vi "Multi-channel FFT(lvgpu).vi"() -> ()   [LabVIEW 2020]
doc: "Computes the 1D FFT of multiple signals simultaneously using a GPU device."
uses:
  subVIs/Channel Data Type.ctl
  <vilib>/addons/lvgpu/lvcufft/CUFFT Type (cufftType).ctl
  <vilib>/addons/lvgpu/lvcufft/Create 1D FFT Plan.vi
  <vilib>/addons/lvgpu/lvcuda/CUDA CSG Device Ptr/Download 2D Data.vi
  <vilib>/addons/lvgpu/lvcufft/Complex FFT (CSG).vi
  <vilib>/addons/lvgpu/lvcuda/CUDA CSG Device Ptr/Upload 2D Data.vi
  <vilib>/addons/lvgpu/lvcufft.lvlib
  <vilib>/addons/lvgpu/lvcuda.lvlib
  subVIs/Multi-channel FFT.lvlib
  <vilib>/ptbypt/NI_PtbyPt.lvlib
  <vilib>/addons/lvgpu/lvcuda/CUDA CSG Device Ptr/CUDA CSG Device Ptr.lvclass
panel:
  in  "Execution Info":T1(tab)
  out "Current Channel":sgl[](graph)
  out "Current Spectrum":sgl[][](graph)
  out "Error Status":errorcluster
  out "CUDA Version":string
  out "CUDA Display Driver Version":string
  out "GPU Device Name":string
  in  "Channel Data":T2 items=["Pulsing Sine Wave", "Fixed Sine Wave", "Drifting Sine Wave"]
  out "GPU Exec Time":dbl format="%#_2p"
  in  "Device ID":i32 min=0 max=0
  out "Intensity Graph (dB)":sgl[][](graph)
  in  "stop":bool
  in  "Samples / channel":i32=1024
  in  "Number of channels":i32=1024
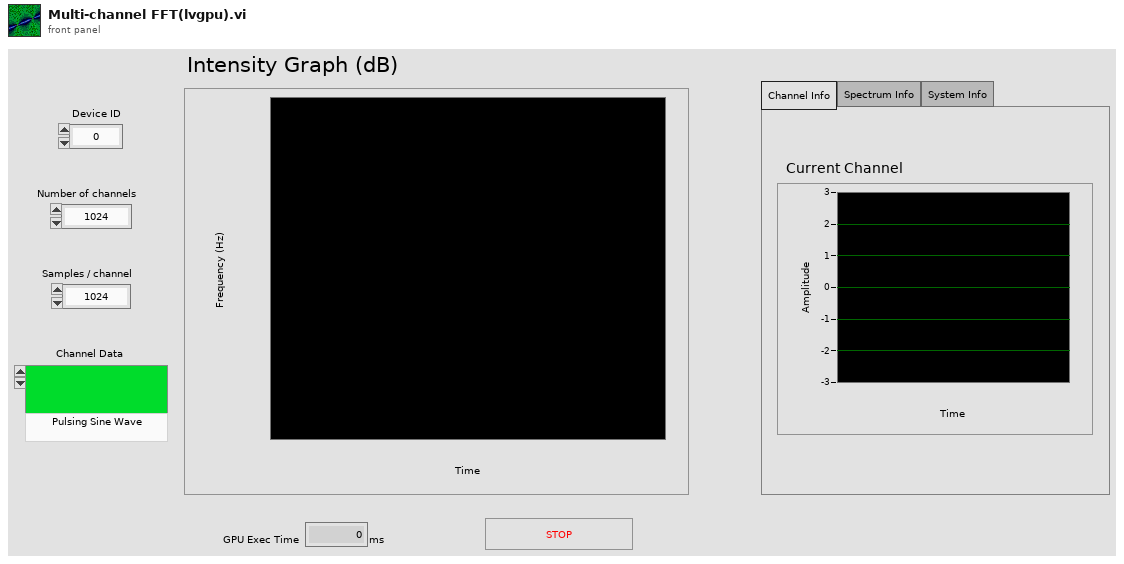
[diagram p1: front panel]
types:
  T1 = enum32{"Channel Info", "Spectrum Info", "System Info"}
  T2 = typedef "Multi-channel FFT.lvlib/Channel Data Type.ctl" = u16
  T3 = typedef "lvcufft.lvlib/CUFFT Type (cufftType).ctl" = i32
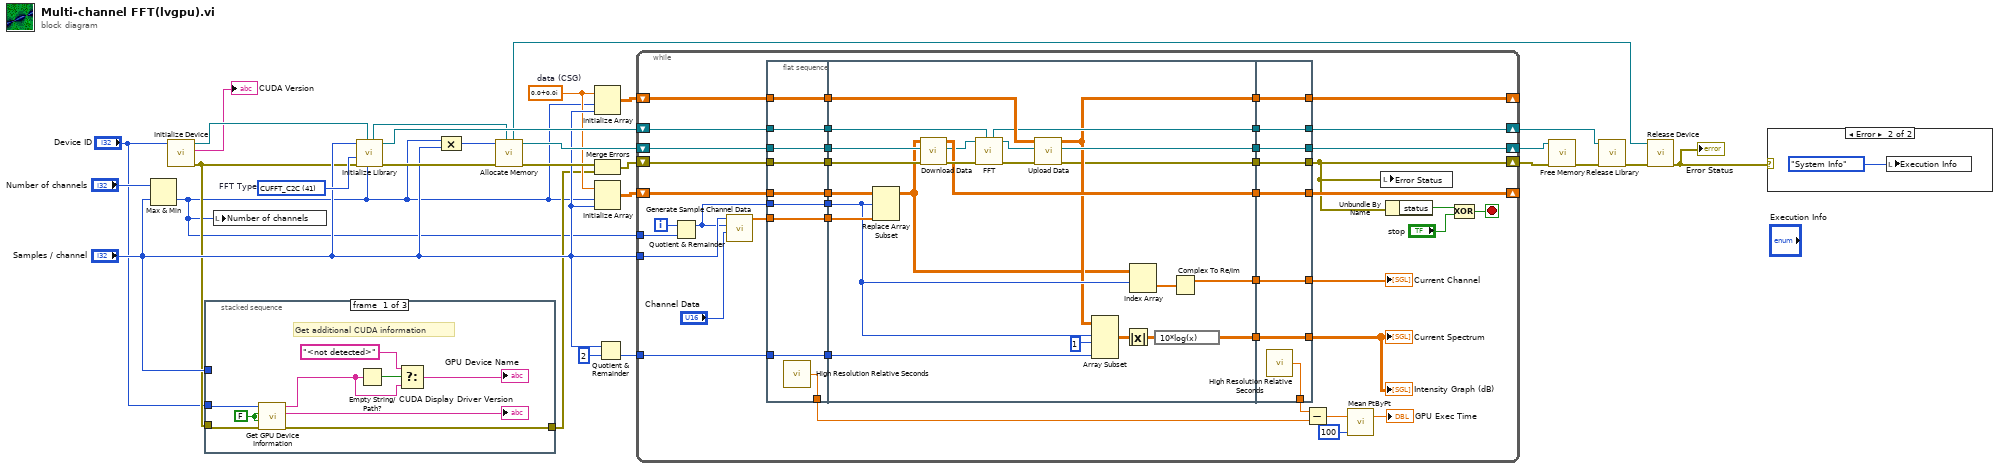
[diagram p0: block diagram]
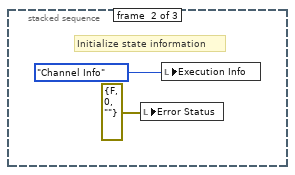
[diagram p3: hidden frame]
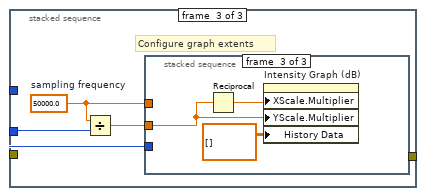
[diagram p4: hidden frame]
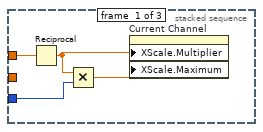
[diagram p5: hidden frame]
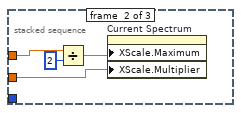
[diagram p6: hidden frame]
diagram:
  w11 = T3 41 items=["CUFFT_R2C"=42, "CUFFT_C2R"=44, "CUFFT_C2C"=41, "CUFFT_D2Z"=106, "CUFFT_Z2D"=108, "CUFFT_Z2Z"=105]  # FFT Type
  w8 = csg 0.0+0.0i  # data (CSG)
  n1 = Max & Min(x="Number of channels", y="Samples / channel") -> (min(x,y)=w1:i32)  [unwired: 1 out]
  n2 = call <vilib>:"Initialize Device.vi"("CUDA Device ID"="Device ID") -> ("error out"=w5:errorcluster, "CUDA Version"=→"CUDA Version":string, "CUDA Context"=w13:refnum<class "CUDA Context.lvclass">)  [unwired: 8 in]
  n3 = stacked-sequence {
    tunnel: "Samples / channel" -> [_ _ w40]
    tunnel: w5 -> [w34 _ _]
    tunnel: "Device ID" -> [w33 _ _]
    tunnel: [w31 _ _] -> w2
    frame #0 {
      w29 = FALSE ("Test Device Execution?")
      # "Get additional CUDA information"
      n4 = call "Get GPU Device Information.vi"("error in"=w34, "Reset Device?"=w29, "Test Device Execution?"=w29, "Device ID"=w33) -> ("error out"=w31:errorcluster, "CUDA Runtime API Version"=→"CUDA Display Driver Version":string, "Device Name"=w32:string)  [unwired: 1 in, 4 out]
      n5 = Empty String/Path?(string/path=w32) -> (empty?=w37:bool)
      n6 = Select(t="<not detected>" ("Name"), s=w37, f=w32) -> (s? t:f=→"GPU Device Name":string)
    }
    frame #1 {
      # "Initialize state information"
      n7 = local write "Error Status"(errorcluster {"status"=FALSE, "code"=0, "source"=""} ("error out")) -> ()
      n8 = local write "Execution Info"(T1."Channel Info" ("Execution Info")) -> ()
    }
    frame #2 {
      w42 = 50000.0  # sampling frequency
      # "Configure graph extents"
      n9 = Divide(x=w42, y=w40) -> (x/y=w41:dbl)
      n10 = stacked-sequence {
        tunnel: w42 -> [w46 w49 _]
        tunnel: w41 -> [_ w50 w51]
        tunnel: w40 -> [w44 _ _]
        frame #0 {
          n11 = Reciprocal(x=w46) -> (1/x=w45:dbl)
          n12 = Multiply(x=w45, y=w44) -> (x*y=w43:dbl)
          n13 = property on="Current Channel" class="WFGraph (strict)"("XScale.Multiplier"=w45, "XScale.Maximum"=w43) -> ()  [unwired: 2 in, 2 out]
        }
        frame #1 {
          n14 = Divide(x=w49, y=2) -> (x/y=w48:dbl)
          n15 = property on="Current Spectrum" class="WFGraph (strict)"("XScale.Maximum"=w48, "XScale.Multiplier"=w50) -> ()  [unwired: 2 in, 2 out]
        }
        frame #2 {
          n16 = Reciprocal(x=w51) -> (1/x=w53:dbl)
          n17 = property on="Intensity Graph (dB)" class="IntChart (strict)"("XScale.Multiplier"=w53, "YScale.Multiplier"=w51, "History Data"=sgl[][] []) -> ()  [unwired: 2 in, 2 out]
        }
      }
    }
  }
  n18 = local write "Number of channels"(w1) -> ()
  n19 = call-poly <vilib>:"Initialize Library.vi"("batch"=w1, "CUDA Context in"=w13, "error in"=w5, "type"=w11, "size"="Samples / channel") -> ("error out"=w15:errorcluster, "CUFFT Handle"=w25:refnum<class "CUFFT Handle.lvclass">, "CUDA Context out"=w12:refnum<class "CUDA Context.lvclass">)  [unwired: 3 in, 1 out]
  n20 = Compound Arithmetic op=MULTIPLY(w1, "Samples / channel") -> (w10:i32)
  n21 = call-poly <vilib>:"Allocate Memory.vi"("CUDA Context in"=w12, "error in"=w15, "size in elements"=w10) -> ("error out"=w17:errorcluster, "CUDA CSG Device Ptr out"=w26:refnum<class "CUDA CSG Device Ptr.lvclass">, "CUDA Context out"=w20:refnum<class "CUDA Context.lvclass">)  [unwired: 6 in]
  n22 = Initialize Array(w8, w1, "Samples / channel") -> (w19:csg[][])
  n23 = Merge Errors(w17, w2) -> (w3:errorcluster)
  n24 = Initialize Array(w8, w1, "Samples / channel") -> (w18:csg[][])
  n25 = Quotient & Remainder(x="Samples / channel", y=2) -> (floor(x/y)=w28:i32)  [unwired: 1 out]
  n26 = while {
    tunnel: w1 -> [w95]
    shift-right: [w83] -> _
    shift-left: w18 -> [w94]
    shift-right: [w76] -> w23
    shift-left: w3 -> [w93]
    tunnel: w28 -> [w91]
    shift-right: [w78] -> _
    shift-left: w19 -> [w92]
    shift-right: [w81] -> w22
    shift-left: w26 -> [w82]
    shift-right: [w88] -> w24
    shift-left: w25 -> [w89]
    tunnel: "Samples / channel" -> [w80]
    i -> [w87]
    stop <- w90 stop-if-true
    n27 = Quotient & Remainder(x=w87, y=w95) -> (x-y*floor(x/y)=w79:i32)  [unwired: 1 out]
    n28 = call "Generate Sample Channel Data.vi"("channel type"="Channel Data", "channel idx"=w79, "sample size"=w80) -> ("channel data"=w86:csg[])  [unwired: 8 in]
    n29 = flat-sequence {
      tunnel: w79 -> [w97]
      tunnel: w82 -> [w98]
      tunnel: w86 -> [w99]
      tunnel: w89 -> [w100]
      tunnel: w91 -> [w101]
      tunnel: w92 -> [w102]
      tunnel: w93 -> [w103]
      tunnel: w94 -> [w104]
      tunnel: [w104] -> w72
      tunnel: [w103] -> w71
      tunnel: [w102] -> w70
      tunnel: [w101] -> w69
      tunnel: [w100] -> w68
      tunnel: [w99] -> w67
      tunnel: [w98] -> w66
      tunnel: [w97] -> w65
      tunnel: [w96] -> w56
      tunnel: w72 -> [w128]
      tunnel: w71 -> [w127]
      tunnel: w70 -> [w126]
      tunnel: w69 -> [w125]
      tunnel: w68 -> [w124]
      tunnel: w67 -> [w122]
      tunnel: w66 -> [w117]
      tunnel: w65 -> [w114]
      tunnel: [w123] -> w64
      tunnel: [w118] -> w63
      tunnel: [w115] -> w62
      tunnel: [w113] -> w61
      tunnel: [w112] -> w60
      tunnel: [w110] -> w59
      tunnel: [w109] -> w58
      tunnel: [w130] -> w74
      tunnel: [w131] -> w75
      tunnel: [w132] -> w76
      tunnel: [w133] -> w78
      tunnel: [w134] -> w81
      tunnel: [w135] -> w83
      tunnel: [w136] -> w88
      tunnel: w64 -> [w136]
      tunnel: w63 -> [w135]
      tunnel: w62 -> [w134]
      tunnel: w61 -> [w133]
      tunnel: w60 -> [w132]
      tunnel: w59 -> [w131]
      tunnel: w58 -> [w130]
      tunnel: [w129] -> w57
      frame #0 {
        n30 = call <vilib>:"High Resolution Relative Seconds.vi"() -> ("relative seconds"=w96:dbl)
      }
      frame #1 {
        n31 = Replace Array Subset(array=w128, new element=w122, index (row)=w114) -> (w106:csg[][])  [unwired: 1 in]
        n32 = call-poly <vilib>:"Download Data.vi"("error in"=w127, "dst in"=w117, "src in"=w106) -> ("error out"=w121:errorcluster, "dst out"=w116:refnum<class "CUDA CSG Device Ptr.lvclass">, "src out"=w118:csg[][])  [unwired: 6 in]
        n33 = call-poly <vilib>:"FFT.vi"("CUFFT Handle in"=w124, "error in"=w121, "signals in"=w116) -> ("error out"=w120:errorcluster, "spectrums out"=w119:refnum<class "CUDA CSG Device Ptr.lvclass">, "CUFFT Handle out"=w123:refnum<class "CUFFT Handle.lvclass">)  [unwired: 6 in]
        n34 = call-poly <vilib>:"Upload Data.vi"("error in"=w120, "src in"=w119, "dst in"=w126) -> ("error out"=w112:errorcluster, "src out"=w115:refnum<class "CUDA CSG Device Ptr.lvclass">, "dst out"=w113:csg[][])  [unwired: 6 in]
        n35 = Array Subset(array=w113, index (row)=w114, length (row)=1 ("length"), length (col)=w125) -> (w107:csg[][])  [unwired: 1 in]
        n36 = Absolute Value(x=w107) -> (abs(x)=w105:sgl[][])
        n37 = Index Array(array=w106, index (row)=w114) -> (element=w111:csg[])  [unwired: 1 in]
        n38 = expression code="10*log(x)"(w105) -> (w109:sgl[][])
        n39 = Complex To Re/Im(x + iy=w111) -> (x=w110:sgl[])  [unwired: 1 out]
      }
      frame #2 {
        n40 = call <vilib>:"High Resolution Relative Seconds.vi"() -> ("relative seconds"=w129:dbl)
      }
    }
    n41 = Subtract(x=w57, y=w56) -> (x-y=w73:dbl)
    n42 = call <vilib>:"Mean PtByPt.vi"("x"=w73, "sample length"=100) -> ("mean"=→"GPU Exec Time":dbl)  [unwired: 2 in, 1 out]
    n43 = local write "Error Status"(w76) -> ()
    n44 = Unbundle By Name(w76) -> ("status"=w85:bool)
    n45 = Compound Arithmetic op=XOR(w85, "stop") -> (w90:bool)
    "Current Channel" <- w75
    "Current Spectrum" <- w74
    "Intensity Graph (dB)" <- w74
  }
  n46 = call-poly <vilib>:"Free Memory.vi"("error in"=w23, "CUDA CSG Device Ptr in"=w22) -> ("error out"=w21:errorcluster)  [unwired: 9 in]
  n47 = call <vilib>:"Release Library.vi"("error in"=w21, "CUFFT Handle in"=w24) -> ("error out"=w27:errorcluster)  [unwired: 9 in]
  n48 = call <vilib>:"Release Device.vi"("error in"=w27, "CUDA Context in"=w20) -> ("error out"=w6:errorcluster)  [unwired: 9 in]
  "Error Status" <- w6
  n49 = case shown="Error" w6 {
    frame No Error {
    }
    frame Error {
      n50 = local write "Execution Info"(T1."System Info" ("Execution Info")) -> ()
    }
  }
